vi "Test 1.vi"(8 "error in (no error)":errorcluster, 11 "Test Case In":refnum<class "Tests.lvclass">) -> (0 "error out":errorcluster, 3 "Test Case Out":refnum<class "Tests.lvclass">)   [LabVIEW 2021, in "Tests.lvclass"]
uses:
  Tests.lvclass
  C:/Program Files (x86)/National Instruments/LabVIEW 2021/vi.lib/Astemes/LUnit/Test Case.lvclass
  <vilib>/Astemes/LUnit/Test Case.lvclass/Test Case.ctl
  4993e8ee-a06a-463a-9684-69129f64d5ce.vi
  <vilib>/Astemes/LUnit/Append Pass Result.vi
  <vilib>/Astemes/LUnit/Append Fail Result.vi
  <vilib>/Astemes/LUnit/Describe Comparison.vi
  <vilib>/Astemes/LUnit/Compare Variants.vi
  <vilib>/Astemes/LUnit/Variant to string.vi
  <vilib>/Utility/Data Type/Get Type Information.vi
  <vilib>/Utility/LVClass/Get LV Class Name.vi
  Proto/Proto.lvclass
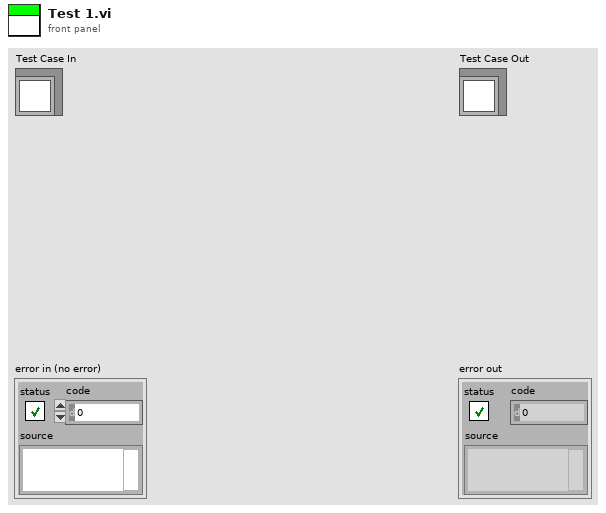
[diagram p1: front panel]
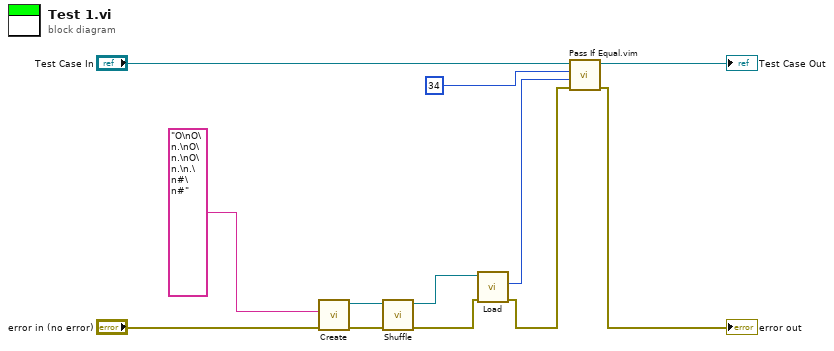
[diagram p0: block diagram]
diagram:
  n1 = call "Create.vi"("error in (no error)"="error in (no error)", "Input"="O\nO\n.\nO\n.\nO\n.\n.\n#\n#") -> ("error out"=w8:errorcluster, "Proto"=w7:refnum<class "Proto.lvclass">)  [unwired: 8 in]
  n2 = call "Shuffle.vi"("error in (no error)"=w8, "Proto in"=w7) -> ("error out"=w5:errorcluster, "Proto out"=w3:refnum<class "Proto.lvclass">)  [unwired: 8 in]
  n3 = call "Load.vi"("error in (no error)"=w5, "Proto in"=w3) -> ("error out"=w4:errorcluster, "Load"=w2:u64)  [unwired: 7 in, 1 out]
  n4 = call "Pass If Equal.vim"("error in (no error)"=w4, "Actual"=w2, "Expected"=u64 34 ("Load"), "LUnit Test Case In"="Test Case In") -> ("error out"=→"error out":errorcluster, "LUnit Test Case Out"=→"Test Case Out":refnum<class "Tests.lvclass">)  [unwired: 6 in]
